vi "Analog Read N Chans.vi"(7 "Analog Ref Override":dbl, 8 "Error In":errorcluster, 10 "AI Channel(s)":u8[](array[numeric]), 11 "LINX Resource":T1) -> (0 "Error Out":errorcluster, 1 "AI Ref":dbl, 2 "Voltages":dbl[](array[numeric]), 3 "LINX Resource":T1)   [LabVIEW 2020, in "LMH-LINX.lvlib"]
doc: "Read the values of the specified analog input channels."
uses:
  LMH-LINX.lvlib
  Private/Type Defs/LINX Ref.ctl
  Private/Type Defs/Platform.ctl
  Private/Type Defs/Interface.ctl
  Private/Device/Type Defs/LINX Device Config.ctl
  Private/Device/Type Defs/TCP Config.ctl
  Private/Device/Type Defs/Channels.ctl
  Private/Type Defs/Peripheral.ctl
  Private/Utilties/Generate Error.vi
  Private/Device/Device.lvlib
  Private/Local IO/Local IO.lvlib
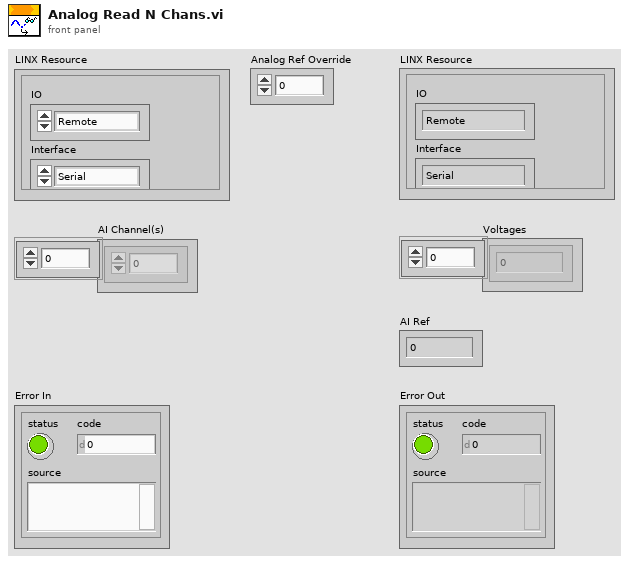
[diagram p1: front panel]
types:
  T1 = typedef "LMH-LINX.lvlib/LINX Ref.ctl" = cluster{"IO":T2, "Interface":T3, "LINX Device Config":T4}
  T2 = typedef "LMH-LINX.lvlib/Platform.ctl" = enum16{"Remote", "Local"}
  T3 = typedef "LMH-LINX.lvlib/Interface.ctl" = enum16{"Serial", "TCP"}
  T4 = typedef "LMH-LINX.lvlib/Device.lvlib/LINX Device Config.ctl" = cluster{"Interface":T3, "COM Port":refnum<visa-resource-name>, "TCP Configuration":T5, "Device Family":u8, "Device ID":u8, "Device Name":string, "TCP Ref":refnum<k5>, "Channels":T6}
  T5 = typedef "LMH-LINX.lvlib/Device.lvlib/TCP Config.ctl" = cluster{"IP Address":string, "Port":u16}
  T6 = typedef "LMH-LINX.lvlib/Channels.ctl" = cluster{"DI":u8[], "DO":u8[], "AI":u8[], "AO":u8[], "PWM":u8[], "QE":u8[], "UART":u8[], "I2C 2":u8[], "SPI":u8[], "CAN":u8[], "Servo":u8[], "AI Ref (V)":dbl, "AI Resolution (Bits)":u8, "AO Ref (V)":dbl, "AO Resolution (Bits)":u8}
  T7 = typedef "LMH-LINX.lvlib/Peripheral.ctl" = enum8{"DI", "DO", "AI", "AO", "PWM", "QE", "UART", "I2C", "SPI", "CAN", "Servo"}
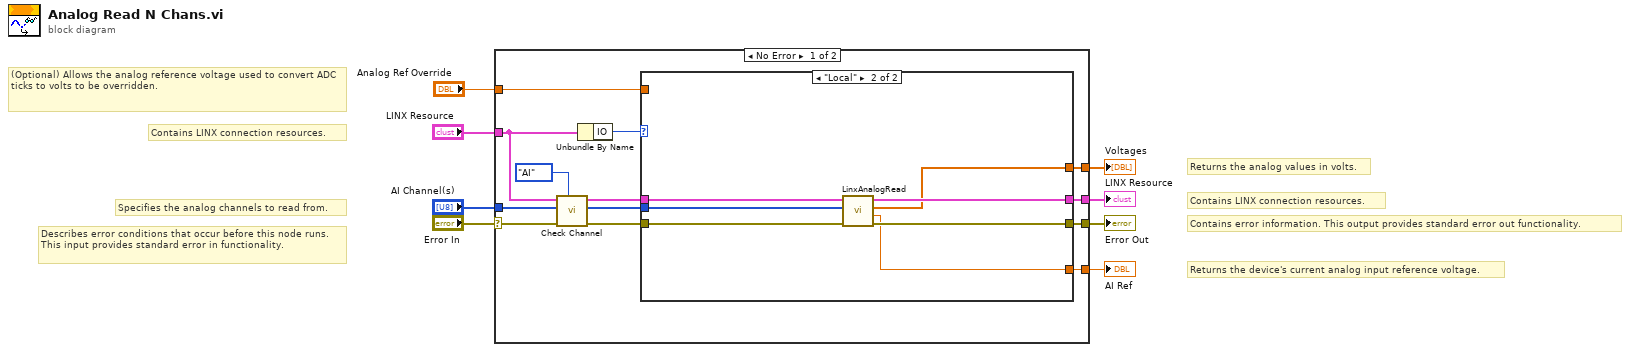
[diagram p0: block diagram]
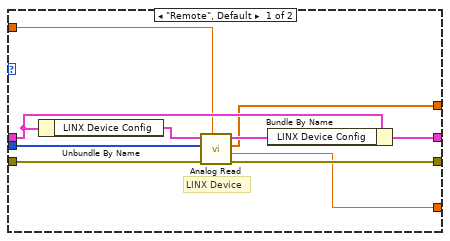
[diagram p2: hidden frame]
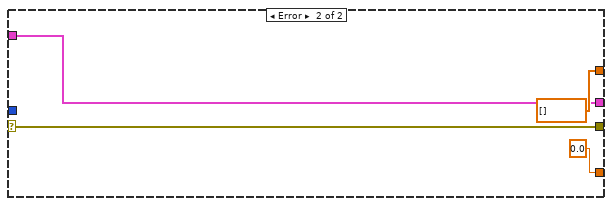
[diagram p3: hidden frame]
diagram:
  # "Returns the analog values in volts."
  # "Returns the device's current analog input reference voltage."
  # "Specifies the analog channels to read from."
  # "(Optional) Allows the analog reference voltage used to convert ADC ticks to volts to be overridden."
  # "Contains LINX connection resources."
  # "Contains error information. This output provides standard error out functionality."
  # "Contains LINX connection resources."
  # "Describes error conditions that occur before this node runs. This input provides standard error in functionality."
  n1 = case shown="No Error" "Error In" {
    selector: "Error In" -> [w11 w42]
    tunnel: [w20 w42] -> w8
    tunnel: [w19 w40] -> w7
    tunnel: "LINX Resource" -> [w9 w40]
    tunnel: "AI Channel(s)" -> [w14 _]
    tunnel: [w13 dbl[] [] ("Values")] -> w4
    tunnel: "Analog Ref Override" -> [w12 _]
    tunnel: [w10 0.0 ("AI Ref")] -> w1
    frame No Error {
      n2 = call "Check Channel.vi"("Peripheral"=Peripheral."AI", "Error In"=w11, "Channels"=w14, "LINX Resource"=w9) -> ("Error Out"=w18:errorcluster, "Channels"=w17:u8[], "LINX Resource"=w15:T1)  [unwired: 5 in]
      n3 = Unbundle By Name(w9) -> ("IO"=w21:T2)
      n4 = case shown="\"Local\"" w21 {
        tunnel: w18 -> [w28 w38]
        tunnel: w15 -> [w31 w37]
        tunnel: [w29 w33] -> w20
        tunnel: [w30 w36] -> w19
        tunnel: w17 -> [w25 w35]
        tunnel: [w24 w34] -> w13
        tunnel: w12 -> [w23 _]
        tunnel: [w22 w32] -> w10
        frame "Remote", Default {
          # "LINX Device"
          n5 = Unbundle By Name(w31) -> ("LINX Device Config"=w27:T4)
          n6 = call "Analog Read.vi"("Analog Ref Override"=w23, "Error In"=w28, "AI Channels"=w25, "LINX Device Config"=w27) -> ("Error Out"=w29:errorcluster, "AI Ref"=w22:dbl, "Voltages"=w24:dbl[], "LINX Device Config"=w26:T4)  [unwired: 4 in]
          n7 = Bundle By Name(cluster=w31, "LINX Device Config"=w26) -> (w30:T1)
        }
        frame "Local" {
          n8 = call "LinxAnalogRead.vi"("Error In"=w38, "Channels"=w35, "LINX Resource"=w37) -> ("Error Out"=w33:errorcluster, "AI Ref"=w32:dbl, "AI Values"=w34:dbl[], "LINX Resource"=w36:T1)  [unwired: 5 in]
        }
      }
    }
    frame Error {
    }
  }
  "Error Out" <- w8
  "LINX Resource" <- w7
  "Voltages" <- w4
  "AI Ref" <- w1
